vi "rdb_net_open.vi"(6 "timeout ms (10000)":i32=10000, 8 "error in (no error)":errorcluster, 10 "port (28015)":u16=28015, 11 "host (\"localhost\")":string="localhost") -> (0 "error out":errorcluster, 3 "conn out":refnum<k5>)   [LabVIEW 2017]
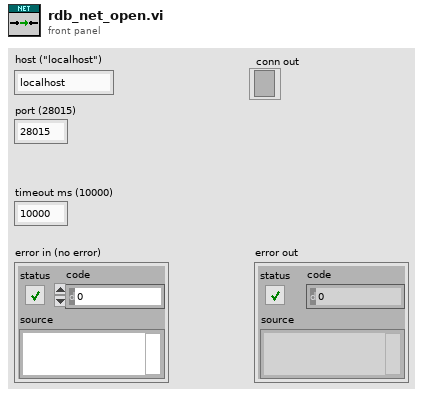
[diagram p1: front panel]
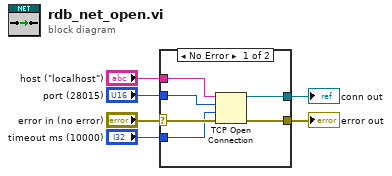
[diagram p0: block diagram]
diagram:
  n1 = case shown="No Error" "error in (no error)" {
    selector: "error in (no error)" -> [w11 w13]
    tunnel: [w12 w13] -> w5
    tunnel: [w10 _] -> w4
    tunnel: "timeout ms (10000)" -> [w9 _]
    tunnel: "host (\"localhost\")" -> [w8 _]
    tunnel: "port (28015)" -> [w7 _]
    frame No Error {
      n2 = TCP Open Connection(address=w8, remote port or service name=w7, timeout ms (60000)=w9, error in (no error)=w11) -> (connection ID=w10:refnum<k5>, error out=w12:errorcluster)  [unwired: 1 in]
    }
    frame Error {
    }
  }
  "error out" <- w5
  "conn out" <- w4
